vi "RichToFlatGreeter_req.vi"(5 "OutputClusterType":T1, 11 "InputCluster":T2) -> (3 "OutputCluster":T1)   [LabVIEW 2019, in "Generated_server.lvlib"]
uses:
  Generated_server.lvlib
  Greeter_req.ctl
  Greeter_req_req_oneof/Greeter_req_req_oneof.lvclass
  Greeter_req_Flat.ctl
  Greeter_req_req_oneof/Greeter_req_req_oneof.lvclass/Greeter_req_req_oneof.ctl
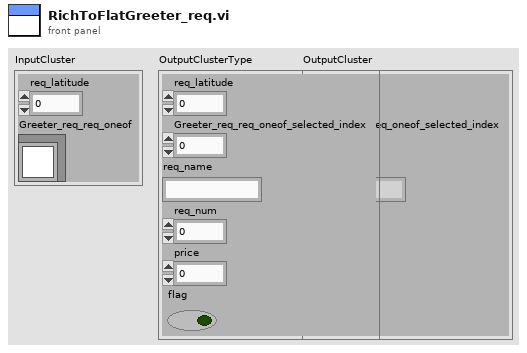
[diagram p1: front panel]
types:
  T1 = typedef "Generated_server.lvlib/Greeter_req_Flat.ctl" = cluster{"req_latitude":i32, "Greeter_req_req_oneof_selected_index":i32, "req_name":string, "req_num":i32, "price":sgl, "flag":bool}
  T2 = typedef "Generated_server.lvlib/Greeter_req.ctl" = cluster{"req_latitude":i32, "Greeter_req_req_oneof":refnum<class "Greeter_req_req_oneof.lvclass">}
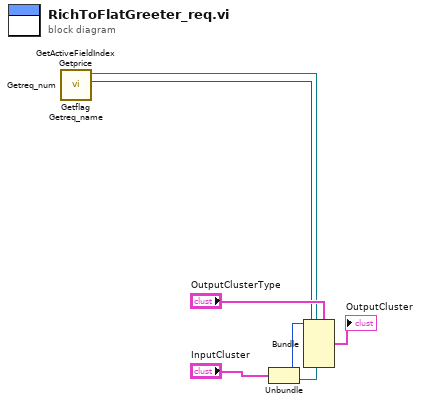
[diagram p0: block diagram]
diagram:
  n1 = Unbundle "Unbundle"("InputCluster") -> ("req_latitude"=w7:i32, "Greeter_req_req_oneof"=w6:refnum<class "Greeter_req_req_oneof.lvclass">)
  n2 = call "Getflag.vi"("OneOfTemplate in"=w6) -> ("Get_Val"=w1:bool)  [unwired: 8 in, 2 out]
  n3 = call "Getprice.vi"("OneOfTemplate in"=w6) -> ("Get_Val"=w2:sgl)  [unwired: 8 in, 2 out]
  n4 = call "Getreq_num.vi"("OneOfTemplate in"=w6) -> ("Get_Val"=w3:i32)  [unwired: 8 in, 2 out]
  n5 = call "Getreq_name.vi"("OneOfTemplate in"=w6) -> ("Get_Val"=w4:string)  [unwired: 8 in, 2 out]
  n6 = call "GetActiveFieldIndex.vi"("OneOfTemplate in"=w6) -> ("Active Field Index"=w5:i32)  [unwired: 8 in, 2 out]
  n7 = Bundle "Bundle"(cluster="OutputClusterType", "req_latitude"=w7, "Greeter_req_req_oneof_selected_index"=w5, "req_name"=w4, "req_num"=w3, "price"=w2, "flag"=w1) -> (→"OutputCluster":T1)
